vi "ke37xx Channel Read.vi"(0 "VISA Resource Name":refnum<visa-resource-name>, 1 "Reading Buffer Name":string, 5 "Channel":string, 7 "Width (1)":u8=1 min=1 max=4 step=1, 9 "Enable Reading Buffer (False)":bool, 11 "error in (no error)":errorcluster) -> (4 "VISA Resource Name Out":refnum<visa-resource-name>, 8 "Data Output":string, 15 "error out":errorcluster)   [LabVIEW 2009, in "Keithley 3700 Series.lvlib"]
doc: "This VI allows reading values from the DAC, totalizer and Digital I/O channels."
uses:
  <instrlib>/Keithley 3706/Keithley 3700 Series.lvlib
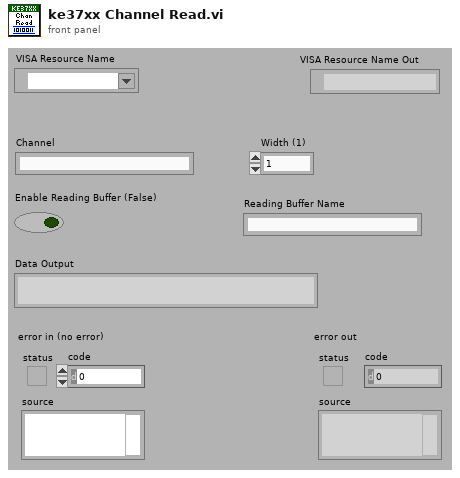
[diagram p1: front panel]
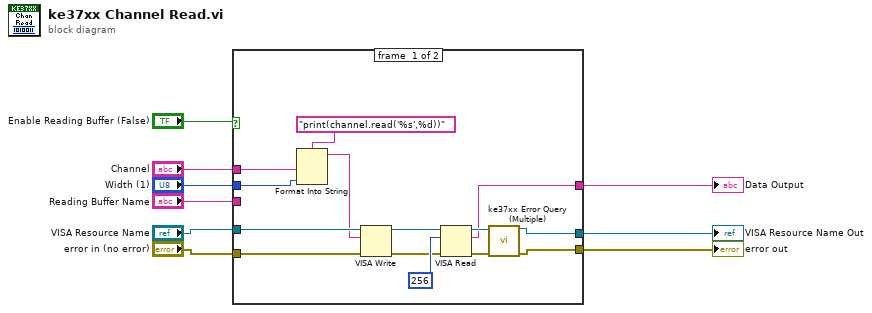
[diagram p0: block diagram]
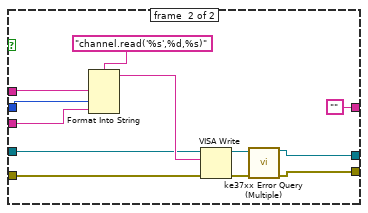
[diagram p2: hidden frame]
diagram:
  n1 = case shown="True" "Enable Reading Buffer (False)" {
    tunnel: "Channel" -> [w23 w34]
    tunnel: "Width (1)" -> [w21 w33]
    tunnel: "Reading Buffer Name" -> [_ w32]
    tunnel: [w15 w28] -> w5
    tunnel: [w14 w27] -> w4
    tunnel: "VISA Resource Name" -> [w13 w26]
    tunnel: "error in (no error)" -> [w12 w25]
    tunnel: [w10 ""] -> w1
    frame #0 {
      n2 = Format Into String(format string="print(channel.read('%s',%d))", w23, w21) -> (resulting string=w11:string)  [unwired: 2 in, 1 out]
      n3 = VISA Write(VISA resource name=w13, write buffer=w11, error in (no error)=w12) -> (VISA resource name out=w19:refnum<visa-resource-name>, error out=w18:errorcluster)  [unwired: 1 out]
      n4 = VISA Read(VISA resource name=w19, byte count=256, error in (no error)=w18) -> (VISA resource name out=w17:refnum<visa-resource-name>, read buffer=w10:string, error out=w16:errorcluster)  [unwired: 1 out]
      n5 = call <instrlib>:"ke37xx Error Query (Multiple).vi"("VISA resource name"=w17, "error in (no error)"=w16) -> ("VISA resource name out"=w15:refnum<visa-resource-name>, "error out"=w14:errorcluster)  [unwired: 12 out]
    }
    frame #1 {
      n6 = Format Into String(format string="channel.read('%s',%d,%s)", w34, w33, w32) -> (resulting string=w29:string)  [unwired: 2 in, 1 out]
      n7 = VISA Write(VISA resource name=w26, write buffer=w29, error in (no error)=w25) -> (VISA resource name out=w31:refnum<visa-resource-name>, error out=w30:errorcluster)  [unwired: 1 out]
      n8 = call <instrlib>:"ke37xx Error Query (Multiple).vi"("VISA resource name"=w31, "error in (no error)"=w30) -> ("VISA resource name out"=w28:refnum<visa-resource-name>, "error out"=w27:errorcluster)  [unwired: 12 out]
    }
  }
  "VISA Resource Name Out" <- w5
  "error out" <- w4
  "Data Output" <- w1
